vi "Send Start Command.vi"(7 "Message Priority (Normal)":T1=enum."Normal", 8 "error in (no error)":errorcluster, 10 "Robot Actors.lvlib:Command.lvlib:Command.lvclass":refnum<class "Command Actor.lvclass">, 11 "Message Enqueuer":refnum<class "Message Enqueuer.lvclass">) -> (0 "error out":errorcluster, 2 "Command notifier":refnum<notifier>, 3 "Message Enqueuer out":refnum<class "Message Enqueuer.lvclass">)   [LabVIEW 2014, in "Robot Actor Framework.lvlib" / "System Actor.lvlib" / "Start Command Msg.lvclass"]
doc: "This VI sends the message to an actor."
uses:
  Start Command Msg.lvclass
  <vilib>/ActorFramework/Message Enqueuer/Message Enqueuer.lvclass
  <vilib>/ActorFramework/Message Enqueuer/Message Priority.ctl
  Command Actor/Command Actor Class/Command Actor.lvclass
  Start Command Msg.lvclass/Start Command Msg.ctl
  <vilib>/ActorFramework/Message Enqueuer/Message Enqueuer.lvclass/Message Enqueuer.ctl
  <vilib>/ActorFramework/Message Priority Queue/Priority Enqueue.vi
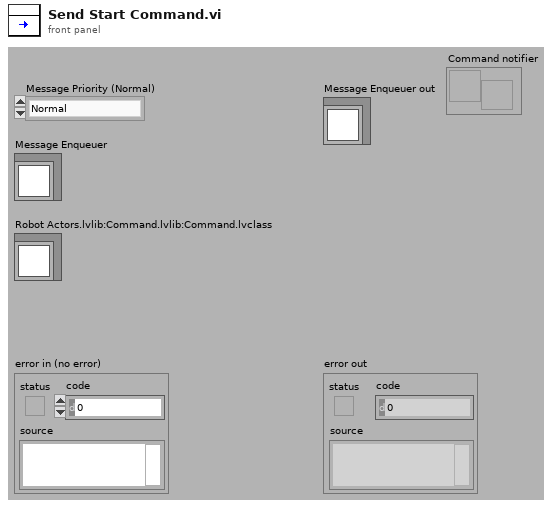
[diagram p1: front panel]
types:
  T1 = typedef "Actor Framework.lvlib/Message Enqueuer.lvclass/Message Priority.ctl" = enum16{"Low", "Normal", "High"}
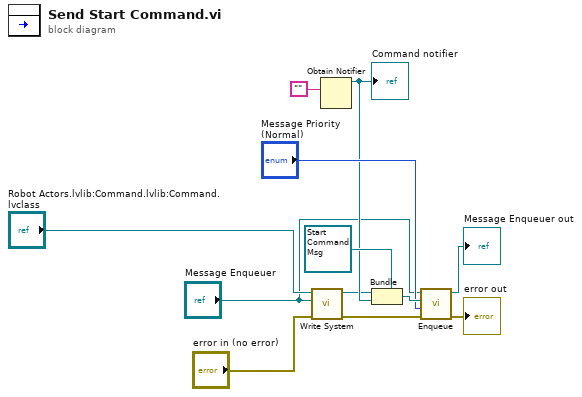
[diagram p0: block diagram]
diagram:
  n1 = call-dynamic "Write System.vi"("error in (no error)"="error in (no error)", "System"="Message Enqueuer", "Command in"="Robot Actors.lvlib:Command.lvlib:Command.lvclass") -> ("error out"=w1:errorcluster, "Command out"=w4:refnum<class "Command Actor.lvclass">)  [unwired: 7 in]
  n2 = Obtain Notifier(notification data type="") -> (notifier out=w6:refnum<notifier>)  [unwired: 3 in, 2 out]
  "Command notifier" <- w6
  n3 = Bundle(cluster=refnum<class "Start Command Msg.lvclass"> refnum ("Object"), w4, w6) -> (w10:refnum<class "Start Command Msg.lvclass">)
  n4 = call <vilib>:"Enqueue.vi"("error in (no error)"=w1, "Message Priority (Normal)"="Message Priority (Normal)", "Message"=w10, "Message Enqueuer in"="Message Enqueuer") -> ("error out"=→"error out":errorcluster, "Message Enqueuer out"=→"Message Enqueuer out":refnum<class "Message Enqueuer.lvclass">)  [unwired: 6 in]
